vi "MALT23T_001_OneCommand_All_Status.vi"   [LabVIEW 2018]
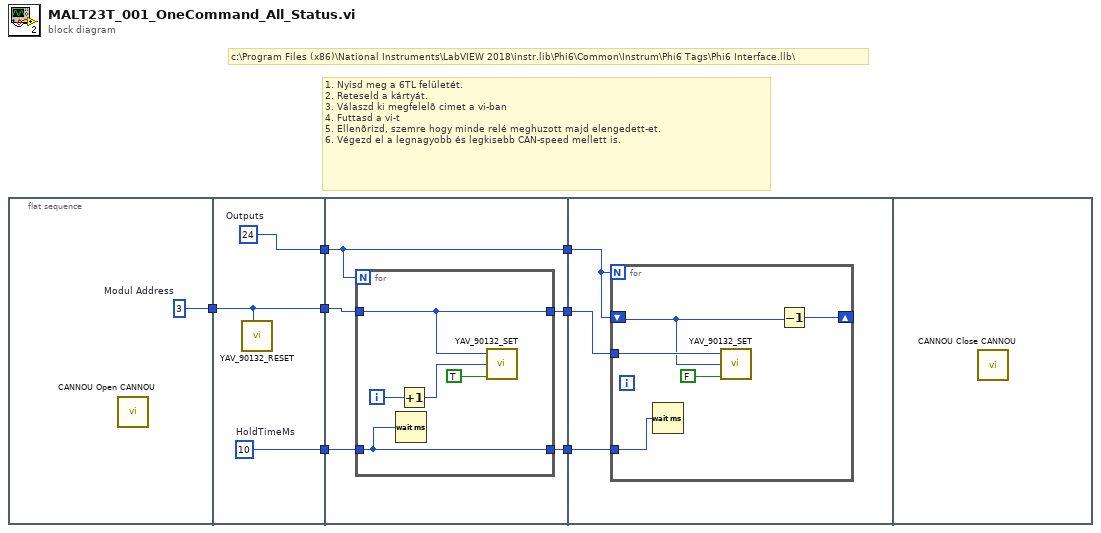
[diagram p0: block diagram]
diagram:
  # "1. Nyisd meg a 6TL felületét.\n2. Reteseld a kártyát.\n3. Válaszd ki megfelelõ cimet a vi-ban\n4. Futtasd a vi-t\n5. Ellenõrizd, szemre hogy minde relé meghuzott majd elengedett-et.\n6. Végezd el a legnagyobb és legkisebb CAN-speed mellett is."
  # "c:\\Program Files (x86)\\National Instruments\\LabVIEW 2018\\instr.lib\\Phi6\\Common\\Instrum\\Phi6 Tags\\Phi6 Interface.llb\\"
  n1 = flat-sequence {
    tunnel: [w8] -> w6
    tunnel: [w11] -> w7
    tunnel: w6 -> [w11]
    tunnel: [w10] -> w5
    tunnel: [w9] -> w3
    tunnel: w7 -> [w16]
    tunnel: w5 -> [w15]
    tunnel: [w15] -> w4
    tunnel: w3 -> [w14]
    tunnel: [w13] -> w2
    tunnel: [w12] -> w1
    tunnel: w4 -> [w24]
    tunnel: w2 -> [w23]
    tunnel: w1 -> [w22]
    frame #0 {
      w8 = u8 3  # Modul Address
      n2 = call <instrlib>:"CANNOU Open CANNOU.vi"() -> ()  [unwired: 6 in, 2 out]
    }
    frame #1 {
      w9 = 10  # HoldTimeMs
      w10 = 24  # Outputs
      n3 = call "YAV_90132_RESET.vi"("Address"=w11) -> ()  [unwired: 4 in, 1 out]
    }
    frame #2 {
      n4 = for {
        N: w15 -> [_]
        tunnel: w16 -> [w17]
        tunnel: w14 -> [w18]
        tunnel: [w18] -> w13
        tunnel: [w17] -> w12
        i -> [w20]
        n5 = Wait (ms)(milliseconds to wait=w18) -> ()  [unwired: 1 out]
        n6 = Increment(x=w20) -> (x+1=w19:i32)
        n7 = call "YAV_90132_SET.vi"("Address"=w17, "Relay Num"=w19, "State"=TRUE) -> ()  [unwired: 2 in, 1 out]
      }
    }
    frame #3 {
      n8 = for {
        N: w24 -> [_]
        shift-right: [w28] -> _
        shift-left: w24 -> [w25]
        tunnel: w23 -> [w27]
        tunnel: w22 -> [w26]
        n9 = Wait (ms)(milliseconds to wait=w27) -> ()  [unwired: 1 out]
        n10 = call "YAV_90132_SET.vi"("Address"=w26, "Relay Num"=w25, "State"=FALSE) -> ()  [unwired: 2 in, 1 out]
        n11 = Decrement(x=w25) -> (x-1=w28:i32)
      }
    }
    frame #4 {
      n12 = call <instrlib>:"CANNOU Close CANNOU.vi"() -> ()  [unwired: 7 in, 1 out]
    }
  }
